vi "PH_ImageOperator.write PSDB Energy data.vi"(0 "i ref in":refnum<vi>, 5 "error in":errorcluster) -> (14 "i ref out":refnum<vi>, 16 "Energy Boolean data":T1[](array[typedef]), 17 "Energy Numeric data":T3[](array[typedef]), 18 "Energy String data":T2[](array[typedef]), 19 "error out":errorcluster)   [LabVIEW 2014, in "PH_ImageOperator.lvlib"]
uses:
  PH_ImageOperator.lvlib
  PH_Basics/PH_PSDBWriter/PH_PSDBWriter.Numeric dataset.ctl
  PH_Basics/PH_PSDBWriter/PH_PSDBWriter.String dataset.ctl
  PH_Basics/PH_PSDBWriter/PH_PSDBWriter.Boolean dataset.ctl
  PH_Basics/PH_PSDBWriter/PH_PSDBWriter.lvlib
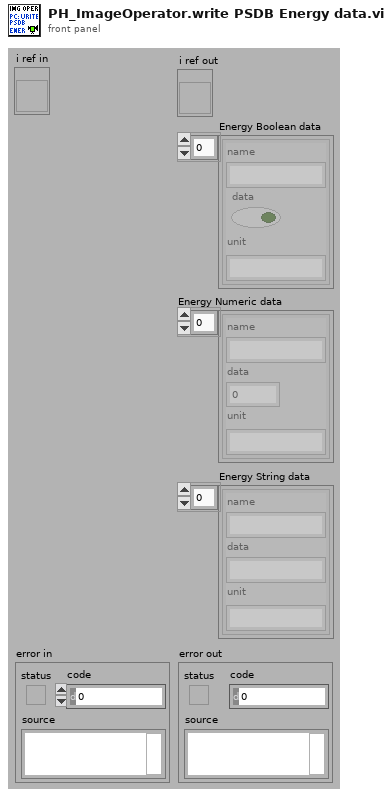
[diagram p1: front panel]
types:
  T1 = typedef "PH_PSDBWriter.lvlib/PH_PSDBWriter.Boolean dataset.ctl" = cluster{"name":string, "data":bool, "unit":string}
  T2 = typedef "PH_PSDBWriter.lvlib/PH_PSDBWriter.String dataset.ctl" = cluster{"name":string, "data":string, "unit":string}
  T3 = typedef "PH_PSDBWriter.lvlib/PH_PSDBWriter.Numeric dataset.ctl" = cluster{"name":string, "data":dbl, "unit":string}
  T4 = typedef "PH_ImageOperator.lvlib/PH_ImageOperator.i attribute.ctl" = cluster{"GUI Refs":cluster{"Delete":refnum<vi>, "Calibration status":refnum<vi>, "BI subtracted":refnum<vi>, "calc Energy":refnum<vi>, "Energy: expected value":refnum<vi>, "Energy: Tolerance":refnum<vi>, "Energy calculated":refnum<vi>, "Energy":refnum<vi>, "calc Beam Anal":refnum<vi>, "Maj Diam 1/esquare":refnum<vi>, "Min Diam 1/esquare":refnum<vi>, "Azi Angle":refnum<vi>, "Min/Maj Diam esquare":refnum<vi>, "Beam analysed":refnum<vi>, "CoG - x":refnum<vi>, "CoG - y":refnum<vi>, "BA: Method":refnum<vi>, "BA: Steps":refnum<vi>, "BA: Factor":refnum<vi>, "calc Traces":refnum<vi>, "Traces: Fit Gauss":refnum<vi>, "Traces calculated":refnum<vi>, "Maj FWHM":refnum<vi>, "Min FWHM":refnum<vi>, "Major Trace":refnum<vi>, "Minor Trace":refnum<vi>, "Maj Fit Order":refnum<vi>, "Min Fit Order":refnum<vi>, "Position calculated":refnum<vi>, "Position":refnum<vi>, "Type":refnum<vi>, "Center":refnum<vi>, "exp - X":refnum<vi>, "exp - Y":refnum<vi>, "Tolerance":refnum<vi>, "f":refnum<vi>, "M":refnum<vi>, "D":refnum<vi>, "q":refnum<vi>, "Dummy Method":refnum<vi>, "Dummy Type":refnum<vi>, "Global On":refnum<vi>, "Traces: No offset":refnum<vi>, "Maj 99%":refnum<vi>, "Min 99%":refnum<vi>, "GUI FF Image":refnum<vi>, "calc Fill Factor":refnum<vi>, "FF calculated":refnum<vi>, "Fill Factor: Filter?":refnum<vi>, "FF: Damage Threshold":refnum<vi>, "FF: Threshold":refnum<vi>, "FF: max allow. Energy":refnum<vi>, "FF: Fillfactor":refnum<vi>, "Calibration data":refnum<vi>}, "List of GUIs":string[], "Calibration":cluster{"Status":T5, "Calibration data":T6, "Calibration Data File":path}, "Final Image":cluster{"BI Subtraction Failure":bool}, "Energy":cluster{"on":bool, "expected value [mJ]":dbl, "Tolerance [%]":dbl, "State":T5, "Energy [mJ]":dbl, "Unit":string, "calculated @":timestamp}, "Beam Analysis":cluster{"on":bool, "Data":T7, "Method":bool, "Steps":i32, "Factor":i32, "ROI":cluster{"Left":i32, "Top":i32, "Right":i32, "Bottom":i32}, "analysed @":timestamp}, "Trace Analysis":cluster{"on":bool, "Fit on":bool, "Maj FWHM":dbl, "Min FWHM":dbl, "Maj Fit Order":i32, "Min Fit Order":i32, "No Offset":bool, "Maj 99%":dbl, "Min 99%":dbl, "Traces":cluster{"XScaleName":string, "Y Scale Minimum":sgl, "Y Scale Maximum":sgl, "X Scale Minimum":sgl, "X Scale Maximum":sgl, "Traces":cluster{"Index":sgl[], "Trace":dbl[]}[]}[], "analysed @":timestamp}, "Position Analysis":cluster{"on":bool, "exp - X":i32, "exp - Y":i32, "focal length [mm]":dbl, "Magnification":dbl, "Delta":dbl, "Theta":dbl, "Tolerance":dbl, "Type":bool, "analysed @":timestamp}, "Fill Factor":cluster{"on":bool, "Filter on?":bool, "Threshold":dbl, "Damage Threshold [J/cm²]":dbl, "Fillfactor":dbl, "Max. allowed Energy [J]":dbl, "calculated @":timestamp}, "Statistician Service ID":i32, "Images":cluster{"Background":T8, "OP":T8, "GUI":T8, "BA: ROI":T8, "Trace: Turn":T8, "FF: Main":T8, "FF: Help":T8, "PSDB: BG":T8, "PSDB: OP":T8, "PSDB: FF":T8}}
  T5 = typedef "PH_StatusHandler.lvlib/PH_StatusHandler.Status.ctl" = i16
  T6 = typedef "PH_ImageCalibrator.lvlib/PH_ImageCalibrator.Calibration Data.ctl" = cluster{"Date":string, "Time":string, "Cam Settings":cluster{"Cam ID":string, "Gain":dbl, "Brightness":dbl, "Shutter":dbl, "Cam Error":bool, "Mode":i32}, "Background Image":cluster{"Image":dbl[][], "Image Error":bool}, "Linear Calibration":cluster{"Calibration Factor":dbl, "not mm or mrad":bool}, "Energy Calibration":cluster{"Calibration Factor":dbl, "no mJ":bool}}
  T7 = typedef "PH_ImageOperator.lvlib/PH_ImageOperator.Beam Analysis Data.ctl" = cluster{"CoG-x":sgl, "CoG-y":sgl, "Maj Dim":dbl, "Min Dim":dbl, "Ellipticity":dbl, "Azimuth Angle [rad]":dbl, "Azi Angle rel to Maj?":bool}
  T8 = typedef "IMAQ Image.ctl" = refnum<image>
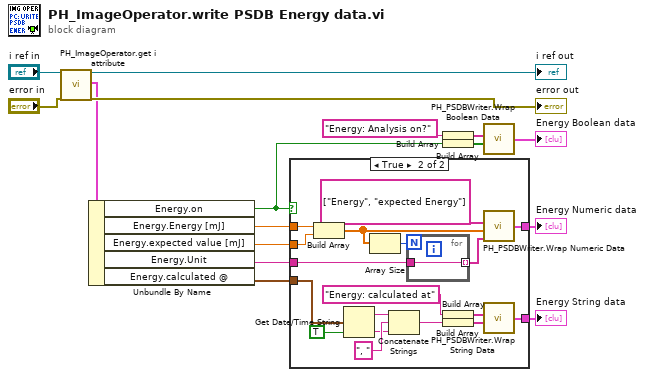
[diagram p0: block diagram]
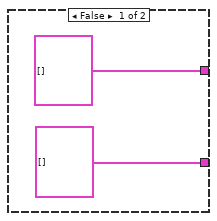
[diagram p2: hidden frame]
diagram:
  n1 = call "PH_ImageOperator.get i attribute.vi"("i ref in"="i ref in", "error in (no error)"="error in") -> ("i ref out"=→"i ref out":refnum<vi>, "i attribute"=w11:T4, "error out"=→"error out":errorcluster)  [unwired: 15 in]
  n2 = Unbundle By Name(w11) -> ("Energy.on"=w5:bool, "Energy.Energy [mJ]"=w10:dbl, "Energy.expected value [mJ]"=w8:dbl, "Energy.Unit"=w9:string, "Energy.calculated @"=w7:timestamp)
  n3 = case shown="True" w5 {
    tunnel: [T3[] [] w28] -> w12
    tunnel: w10 -> [_ w36]
    tunnel: w9 -> [_ w27]
    tunnel: w8 -> [_ w35]
    tunnel: w7 -> [_ w30]
    tunnel: [T2[] [] w23] -> w6
    frame False {
    }
    frame True {
      n4 = Build Array(w36, w35) -> (w24:dbl[])
      n5 = Get Date/Time String(seconds (now)=w30, want seconds? (F)=TRUE) -> (date string=w33:string, time string=w31:string)  [unwired: 1 in]
      n6 = Array Size(array=w24) -> (size(s)=w25:i32)
      n7 = Concatenate Strings(w33, ", " ("string"), w31) -> (w21:string)
      n8 = for {
        N: w25 -> [_]
        tunnel: w27 -> [w37]
        tunnel: [w37] -> w26 mode=indexing
      }
      n9 = Build Array("Energy: calculated at" ("name")) -> (w19:string[])
      n10 = Build Array(w21) -> (w20:string[])
      n11 = call "PH_PSDBWriter.Wrap Numeric Data.vi"("Unit Array"=w26, "Data Array"=w24, "Name Array"=string[] ["Energy", "expected Energy"]) -> ("PSDB Numeric Data Array"=w28:T3[])  [unwired: 1 in]
      n12 = call "PH_PSDBWriter.Wrap String Data.vi"("Data Array"=w20, "Name Array"=w19) -> ("PSDB String Data Array"=w23:T2[])  [unwired: 2 in]
    }
  }
  "Energy Numeric data" <- w12
  "Energy String data" <- w6
  n13 = Build Array("Energy: Analysis on?" ("name")) -> (w1:string[])
  n14 = Build Array(w5) -> (w2:bool[])
  n15 = call "PH_PSDBWriter.Wrap Boolean Data.vi"("Data Array"=w2, "Name Array"=w1) -> ("PSDB Boolean Data Array"=→"Energy Boolean data":T1[])  [unwired: 2 in]
